vi "Configure RemIO Module Core.vi"(8 "error in (no error)":errorcluster, 9 "module slot index":u8=1, 10 "Slave Ref In":refnum<k21>, 11 "11120 in":refnum<class "11120.lvclass">) -> (0 "error out":errorcluster, 1 "negative confirmation":T1 {"additional error code" format="%.0x"; "error code" format="%.0x"}, 2 "Slave Ref Out":refnum<k21>, 3 "11120 out":refnum<class "11120.lvclass">, 5 "SDO abort code":u32 format="%.0x")   [LabVIEW 2019, in "Modules.lvlib" / "11120.lvclass"]
uses:
  11120.lvclass
  <vilib>/indcomecat/Remote IO/typedefs/negative confirmation.ctl
  11120.lvclass/11120.ctl
  3882c9f9-c922-4739-ba2d-1f6f080df7b6.vi
  RemIO Module/Get RemIO Library Path.vi
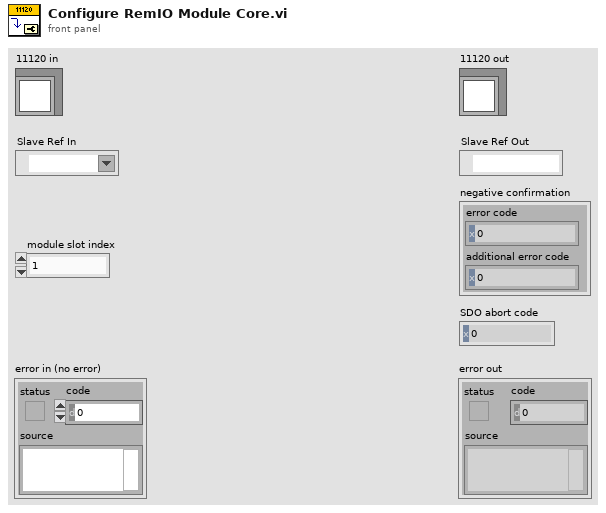
[diagram p1: front panel]
types:
  T1 = typedef "negative confirmation.ctl" = cluster{"error code":u16, "additional error code":u16}
  T2 = typedef "NI ECAT Remote IO.lvlib/mounting position REM-11120.ctl" = u8
  T3 = typedef "NI ECAT Remote IO.lvlib/channel number REM-11120.ctl" = u8
  T4 = typedef "NI ECAT Remote IO.lvlib/input filter time REM-11120.ctl" = u8
  T5 = typedef "NI ECAT Remote IO.lvlib/cold junction type REM-11120.ctl" = u8
  T6 = typedef "NI ECAT Remote IO.lvlib/resolution REM-11120.ctl" = u8
  T7 = typedef "NI ECAT Remote IO.lvlib/sensor type REM-11120.ctl" = u8
  T8 = cluster{"mounting position":T2, "parameters for channels":cluster{"channel number":T3, "input filter time":T4, "cold junction type":T5, "resolution":T6, "sensor type":T7}[]}
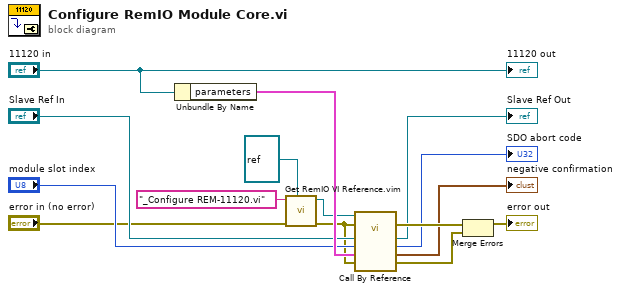
[diagram p0: block diagram]
diagram:
  n1 = Unbundle By Name("11120 in") -> ("parameters"=w12:T8)
  n2 = call "Get RemIO VI Reference.vim"("name or relative path"="_Configure REM-11120.vi", "error in (no error)"="error in (no error)", "type specifier VI Refnum (for type only)"=refnum<vi> refnum) -> ("vi reference"=w1:refnum<vi>, "error out"=w4:errorcluster)  [unwired: 6 in]
  n3 = call-by-ref "?"(reference=w1, error in=w4, 8:"error in (no error)"=w4, "parameters"=w12, "module slot index"="module slot index", "slave reference in"="Slave Ref In") -> (error out=w13:errorcluster, 0:"error out"=w14:errorcluster, "negative confirmation"=→"negative confirmation":T1, "SDO abort code"=→"SDO abort code":u32, "slave reference out"=→"Slave Ref Out":refnum<k21>)  [unwired: 4 in, 1 out]
  n4 = Merge Errors(w13, w14) -> (→"error out":errorcluster)
  "11120 out" <- "11120 in"
